vi "ex6.vi"() -> ()   [LabVIEW 2020]
panel:
  in  "Boolean":bool
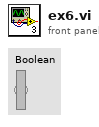
[diagram p1: front panel]
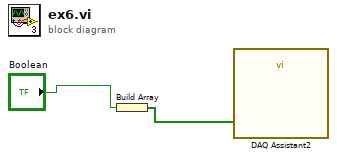
[diagram p0: block diagram]
diagram:
  n1 = Build Array("Boolean") -> (w2:bool[])
  n2 = call "DAQ Assistant2"("data"=w2) -> ()  [unwired: 17 in, 2 out]
